vi "ACS712.vi"(11 "ACS712":dbl[](array[numeric]) format="%.4f") -> (3 "Current":dbl)   [LabVIEW 2018, in "Test_Libraries.lvlib"]
uses:
  Proyecto/Test_Libraries.lvlib
  <vilib>/Analysis/NI_AALPro.lvlib
  <vilib>/Analysis/5stat.llb/RMS (DBL).vi
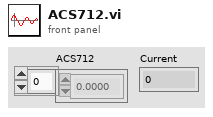
[diagram p1: front panel]
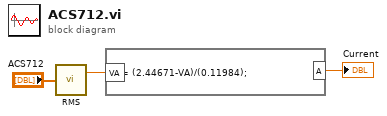
[diagram p0: block diagram]
diagram:
  n1 = call-poly <vilib>:"RMS.vi"("X"="ACS712") -> ("rms value"=w3:dbl)  [unwired: 1 out]
  n2 = formula code="A= (2.44671-VA)/(0.11984);"("VA"=w3) -> ("A"=→"Current":dbl)
